vi "Match Key Regex.vi"(8 "error in":errorcluster, 10 "Datatype":T1, 11 "key in":string) -> (0 "error out":errorcluster, 1 "Datatype Found?":bool, 2 "Label out":string, 3 "key out":string)   [LabVIEW 2019, in "Instrument.Lockin.lvlib" / "Instrument.Lockin.lvclass"]
uses:
  Instrument.Lockin.lvclass
  Typedefs/Results Type--Enum.ctl
  <vilib>/regexp/Match Regular Expression.xnode
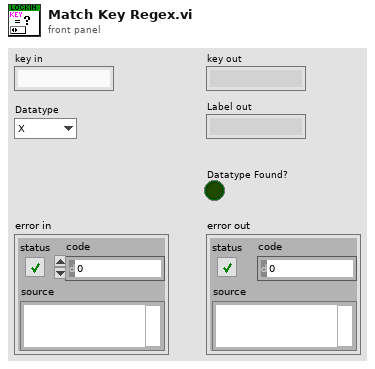
[diagram p1: front panel]
types:
  T1 = typedef "Instrument.Lockin.lvlib/Instrument.Lockin.lvclass/Results Type--Enum.ctl" = enum16{"X", "Y", "R", "Theta", "Mean"}
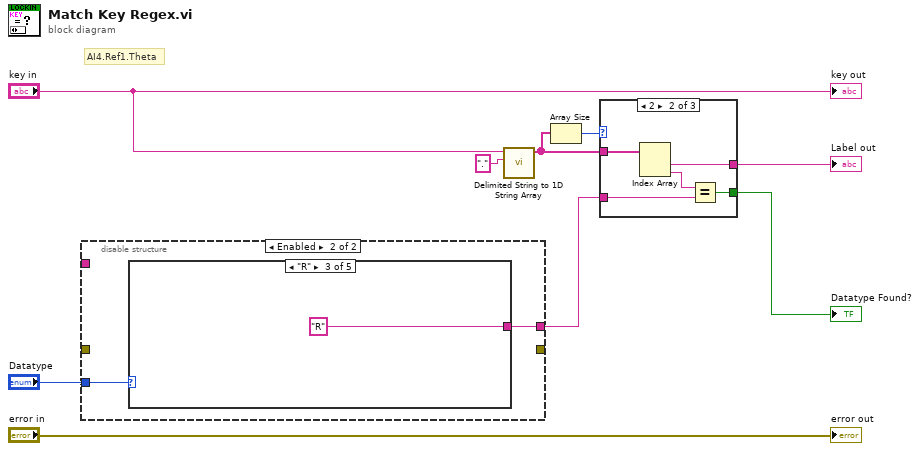
[diagram p0: block diagram]
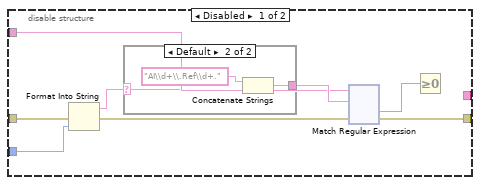
[diagram p2: hidden frame]
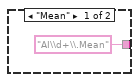
[diagram p3: hidden frame]
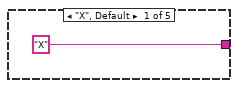
[diagram p4: hidden frame]
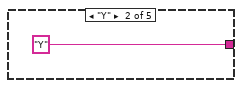
[diagram p5: hidden frame]
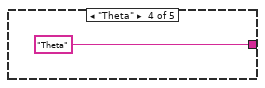
[diagram p6: hidden frame]
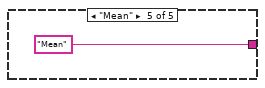
[diagram p7: hidden frame]
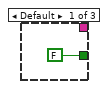
[diagram p8: hidden frame]
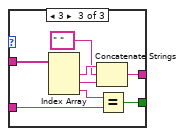
[diagram p9: hidden frame]
diagram:
  # "AI4.Ref1.Theta"
  n1 = disable-structure shown="Enabled" {
    disable-tunnel: "Datatype" -> [w14 w137]
    disable-tunnel: [w13 _] -> _
    disable-tunnel: _ -> [w12 _]
    disable-tunnel: _ -> [w10 _]
    disable-tunnel: [_ w136] -> w1
    frame Disabled {
      n2 = Format Into String(error in=w12, w14) -> (resulting string=w15:string, error out=w11:errorcluster)  [unwired: 2 in]
      n3 = case shown="Default" w15 {
        selector: w15 -> [_ w20]
        tunnel: ["AI\\d+\\.Mean" ("regular expression") w19] -> w17
        frame "Mean" {
        }
        frame Default {
          n4 = Concatenate Strings("AI\\d+\\.Ref\\d+." ("regular expression"), w20) -> (w19:string)
        }
      }
      n5 = xnode "Match Regular Expression"("input string"=w10, "regular expression"=w17, "error in"=w11) -> ("offset past match"=w16:i32, "error out"=w13:errorcluster)  [unwired: 3 in, 3 out]
      n6 = Greater Or Equal To 0?(x=w16) -> ()  [unwired: 1 out]
    }
    frame Enabled {
      n7 = case shown="\"R\"" w137 {
        tunnel: ["X" ("y") "Y" ("y") "R" ("y") "Theta" ("y") "Mean" ("y")] -> w136
        frame "X", Default {
        }
        frame "Y" {
        }
        frame "R" {
        }
        frame "Theta" {
        }
        frame "Mean" {
        }
      }
    }
  }
  n8 = call <vilib>:"Delimited String to 1D String Array.vi"("delimiter"=".", "delimited string"="key in") -> ("string array"=w6:string[])  [unwired: 9 in]
  n9 = Array Size(array=w6) -> (size(s)=w7:i32)
  n10 = case shown="2" w7 {
    tunnel: w6 -> [_ w148 w156]
    tunnel: [_ w147 w155] -> w5
    tunnel: [FALSE w146 w150] -> w2
    tunnel: w1 -> [_ w145 w151]
    frame Default {
    }
    frame 2 {
      n11 = Index Array(array=w148) -> (element #1=w147:string, element #2=w144:string)  [unwired: 2 in]
      n12 = Equal?(x=w144, y=w145) -> (x = y?=w146:bool)
    }
    frame 3 {
      n13 = Index Array(array=w156) -> (element #1=w154:string, element #2=w152:string, element #3=w149:string)  [unwired: 3 in]
      n14 = Concatenate Strings(w154, " " ("string"), w152) -> (w155:string)
      n15 = Equal?(x=w149, y=w151) -> (x = y?=w150:bool)
    }
  }
  "Datatype Found?" <- w2
  "Label out" <- w5
  "key out" <- "key in"
  "error out" <- "error in"
